vi "EyePositionBin.vi"(7 "bin":i32=10, 8 "gaze Threshold":dbl=75.0, 9 "pupil input":cluster{"Pos. X":dbl, "Pos. Y":dbl}, 10 "CR input":cluster{"Pos. X":dbl, "Pos. Y":dbl}, 11 "data array input":T1) -> (0 "data array output":T2, 1 "gaze":bool, 3 "eyeposition array":dbl[](array[numeric]))   [LabVIEW 2011]
uses:
  <vilib>/Analysis/NI_AALBase.lvlib
panel:
  in  "枚举":enum16{""}(ring)
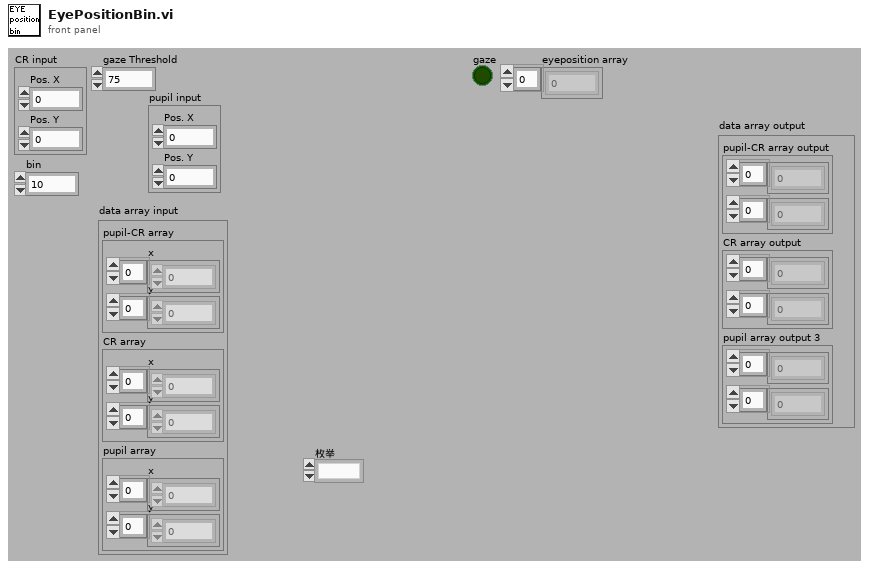
[diagram p1: front panel]
types:
  T1 = cluster{"pupil-CR array":cluster{"x":dbl[], "y":dbl[]}, "CR array":cluster{"x":dbl[], "y":dbl[]}, "pupil array":cluster{"x":dbl[], "y":dbl[]}}
  T2 = cluster{"pupil-CR array output":cluster{dbl[], dbl[]}, "CR array output":cluster{dbl[], dbl[]}, "pupil array output 3":cluster{dbl[], dbl[]}}
  T3 = cluster{cluster{dbl[], dbl[]}, cluster{dbl[], dbl[]}, cluster{dbl[], dbl[]}}
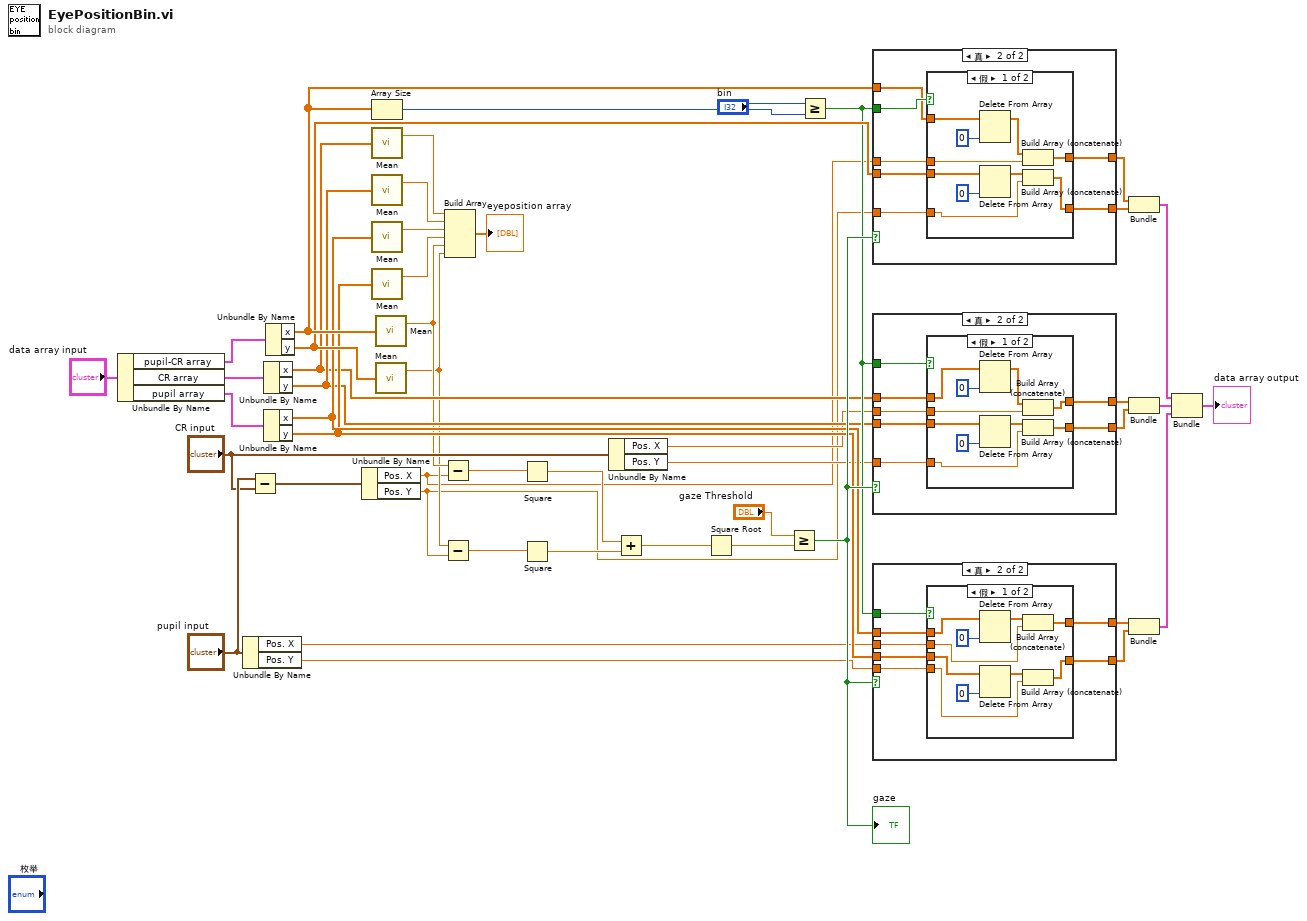
[diagram p0: block diagram]
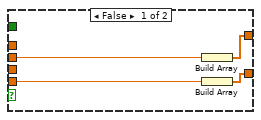
[diagram p2: hidden frame]
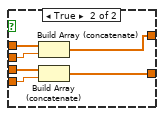
[diagram p3: hidden frame]
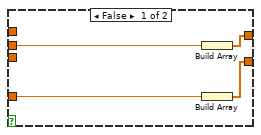
[diagram p4: hidden frame]
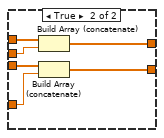
[diagram p5: hidden frame]
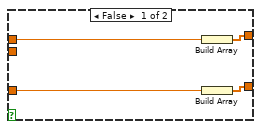
[diagram p6: hidden frame]
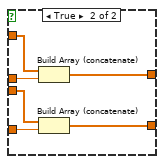
[diagram p7: hidden frame]
diagram:
  n1 = Unbundle By Name("data array input") -> ("pupil-CR array"=w20:cluster{"x":dbl[], "y":dbl[]}, "CR array"=w19:cluster{"x":dbl[], "y":dbl[]}, "pupil array"=w18:cluster{"x":dbl[], "y":dbl[]})
  n2 = Unbundle By Name("pupil input") -> ("Pos. X"=w5:dbl, "Pos. Y"=w4:dbl)
  n3 = Subtract(x="pupil input", y="CR input") -> (x-y=w34:cluster{"Pos. X":dbl, "Pos. Y":dbl})
  n4 = Unbundle By Name(w19) -> ("x"=w12:dbl[], "y"=w13:dbl[])
  n5 = Unbundle By Name(w18) -> ("x"=w17:dbl[], "y"=w16:dbl[])
  n6 = Unbundle By Name(w20) -> ("x"=w36:dbl[], "y"=w35:dbl[])
  n7 = Unbundle By Name(w34) -> ("Pos. X"=w3:dbl, "Pos. Y"=w2:dbl)
  n8 = Array Size(array=w36) -> (size(s)=w47:i32)
  n9 = call <vilib>:"Mean.vi"("X"=w12) -> ("mean"=w9:dbl)  [unwired: 1 out]
  n10 = call <vilib>:"Mean.vi"("X"=w13) -> ("mean"=w8:dbl)  [unwired: 1 out]
  n11 = call <vilib>:"Mean.vi"("X"=w17) -> ("mean"=w15:dbl)  [unwired: 1 out]
  n12 = call <vilib>:"Mean.vi"("X"=w16) -> ("mean"=w14:dbl)  [unwired: 1 out]
  n13 = call <vilib>:"Mean.vi"("X"=w36) -> ("mean"=w11:dbl)  [unwired: 1 out]
  n14 = call <vilib>:"Mean.vi"("X"=w35) -> ("mean"=w10:dbl)  [unwired: 1 out]
  n15 = Subtract(x=w11, y=w3) -> (x-y=w45:dbl)
  n16 = Subtract(x=w10, y=w2) -> (x-y=w44:dbl)
  n17 = Build Array(w9, w8, w15, w14, w11, w10) -> (→"eyeposition array":dbl[])
  n18 = Square(x=w45) -> (x^2=w43:dbl)
  n19 = Square(x=w44) -> (x^2=w42:dbl)
  n20 = Unbundle By Name("CR input") -> ("Pos. X"=w7:dbl, "Pos. Y"=w6:dbl)
  n21 = Add(x=w43, y=w42) -> (x+y=w41:dbl)
  n22 = Square Root(x=w41) -> (sqrt(x)=w39:dbl)
  n23 = Greater Or Equal?(x="gaze Threshold", y=w39) -> (x >= y?=w27:bool)
  "gaze" <- w27
  n24 = Greater Or Equal?(x="bin", y=w47) -> (x >= y?=w26:bool)
  n25 = case shown="真" w27 {
    tunnel: w3 -> [w51 w56]
    tunnel: w2 -> [w50 w54]
    tunnel: [w49 w53] -> w38
    tunnel: [w48 w52] -> w37
    tunnel: w26 -> [_ w58]
    tunnel: w36 -> [_ w57]
    tunnel: w35 -> [_ w55]
    frame False {
      n26 = Build Array(w51) -> (w49:dbl[])
      n27 = Build Array(w50) -> (w48:dbl[])
    }
    frame True {
      n28 = case shown="假" w58 {
        tunnel: w57 -> [w68 w74]
        tunnel: w56 -> [w65 w73]
        tunnel: w55 -> [w63 w72]
        tunnel: w54 -> [w60 w71]
        tunnel: [w64 w70] -> w53
        tunnel: [w59 w69] -> w52
        frame False {
          n29 = Delete From Array(array=w68, index=0 ("索引")) -> (array with subset deleted=w66:dbl[])  [unwired: 1 in, 1 out]
          n30 = Delete From Array(array=w63, index=0 ("索引")) -> (array with subset deleted=w62:dbl[])  [unwired: 1 in, 1 out]
          n31 = Build Array (concatenate)(w66, w65) -> (w64:dbl[])
          n32 = Build Array (concatenate)(w62, w60) -> (w59:dbl[])
        }
        frame True {
          n33 = Build Array (concatenate)(w74, w73) -> (w70:dbl[])
          n34 = Build Array (concatenate)(w72, w71) -> (w69:dbl[])
        }
      }
    }
  }
  n35 = case shown="真" w27 {
    tunnel: w7 -> [w78 w84]
    tunnel: w6 -> [w77 w83]
    tunnel: [w76 w82] -> w30
    tunnel: [w75 w81] -> w31
    tunnel: w26 -> [_ w85]
    tunnel: w12 -> [_ w80]
    tunnel: w13 -> [_ w79]
    frame False {
      n36 = Build Array(w78) -> (w76:dbl[])
      n37 = Build Array(w77) -> (w75:dbl[])
    }
    frame True {
      n38 = case shown="假" w85 {
        tunnel: w84 -> [w94 w101]
        tunnel: w83 -> [w91 w100]
        tunnel: [w93 w99] -> w82
        tunnel: [w90 w98] -> w81
        tunnel: w80 -> [w89 w97]
        tunnel: w79 -> [w88 w96]
        frame False {
          n39 = Delete From Array(array=w89, index=0 ("索引")) -> (array with subset deleted=w87:dbl[])  [unwired: 1 in, 1 out]
          n40 = Delete From Array(array=w88, index=0 ("索引")) -> (array with subset deleted=w86:dbl[])  [unwired: 1 in, 1 out]
          n41 = Build Array (concatenate)(w87, w94) -> (w93:dbl[])
          n42 = Build Array (concatenate)(w86, w91) -> (w90:dbl[])
        }
        frame True {
          n43 = Build Array (concatenate)(w97, w101) -> (w99:dbl[])
          n44 = Build Array (concatenate)(w96, w100) -> (w98:dbl[])
        }
      }
    }
  }
  n45 = case shown="真" w27 {
    tunnel: w5 -> [w105 w111]
    tunnel: w4 -> [w104 w110]
    tunnel: [w103 w109] -> w29
    tunnel: [w102 w108] -> w28
    tunnel: w26 -> [_ w112]
    tunnel: w17 -> [_ w107]
    tunnel: w16 -> [_ w106]
    frame False {
      n46 = Build Array(w105) -> (w103:dbl[])
      n47 = Build Array(w104) -> (w102:dbl[])
    }
    frame True {
      n48 = case shown="假" w112 {
        tunnel: w111 -> [w121 w128]
        tunnel: w110 -> [w118 w127]
        tunnel: [w120 w126] -> w109
        tunnel: [w117 w125] -> w108
        tunnel: w107 -> [w116 w124]
        tunnel: w106 -> [w115 w123]
        frame False {
          n49 = Delete From Array(array=w116, index=0 ("索引")) -> (array with subset deleted=w114:dbl[])  [unwired: 1 in, 1 out]
          n50 = Delete From Array(array=w115, index=0 ("索引")) -> (array with subset deleted=w113:dbl[])  [unwired: 1 in, 1 out]
          n51 = Build Array (concatenate)(w114, w121) -> (w120:dbl[])
          n52 = Build Array (concatenate)(w113, w118) -> (w117:dbl[])
        }
        frame True {
          n53 = Build Array (concatenate)(w124, w128) -> (w126:dbl[])
          n54 = Build Array (concatenate)(w123, w127) -> (w125:dbl[])
        }
      }
    }
  }
  n55 = Bundle(w38, w37) -> (w25:cluster{dbl[], dbl[]})  [unwired: 1 out]
  n56 = Bundle(w30, w31) -> (w24:cluster{dbl[], dbl[]})  [unwired: 1 out]
  n57 = Bundle(w29, w28) -> (w23:cluster{dbl[], dbl[]})  [unwired: 1 out]
  n58 = Bundle(w25, w24, w23) -> (→"data array output":T3)  [unwired: 1 out]
